vi "Calc_Actuators_SP PV to Power.vi"(0 "Power IN":dbl=0.01 format="%#_13g", 3 "Setpoint":dbl format="%.1f", 4 "Process Variable":dbl format="%.1f", 7 "power rate per iter":dbl=0.01 format="%#_13g", 9 "Deadband":dbl=1.0 format="%#_13g", 11 "Limit Max":dbl format="%.1f", 13 "Limit Min":dbl format="%.1f") -> (14 "Power OUT":dbl=0.01 format="%#_13g")   [LabVIEW 2017]
uses:
  Type Definitions/typedef_enum_Actuator Action.ctl
  7370e306-27d6-4c0f-bd38-d504dbee8b0f.vi
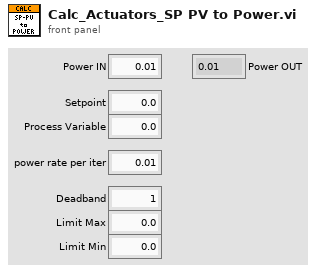
[diagram p1: front panel]
types:
  T1 = typedef "typedef_enum_Actuator Action.ctl" = enum16{"Low Limit", "Deadband", "High Limit", "Retract", "Extend"}
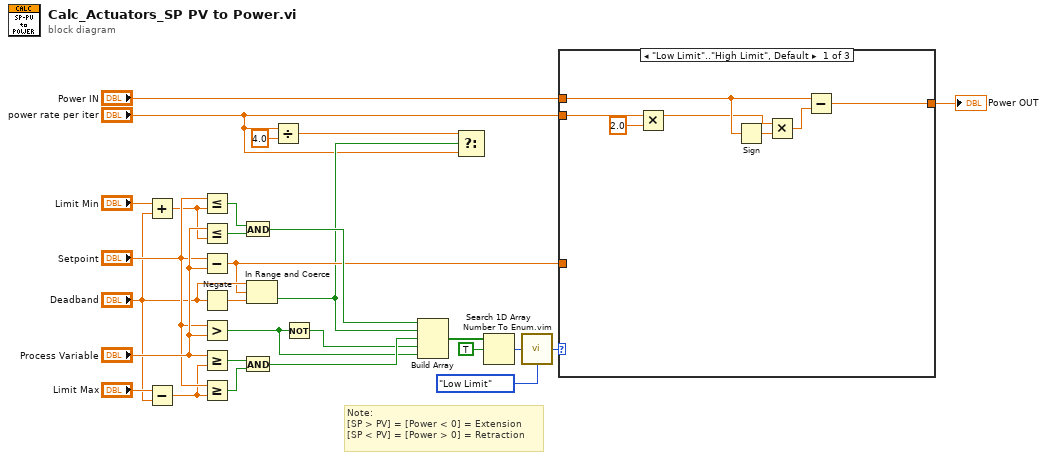
[diagram p0: block diagram]
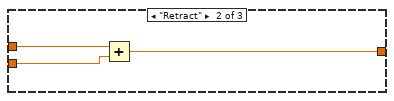
[diagram p2: hidden frame]
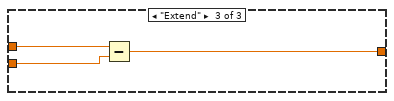
[diagram p3: hidden frame]
diagram:
  # "Note:\n[SP > PV] = [Power < 0] = Extension\n[SP < PV] = [Power > 0] = Retraction"
  n1 = Add(x="Limit Min", y="Deadband") -> (x+y=w10:dbl)
  n2 = Subtract(x="Limit Max", y="Deadband") -> (x-y=w11:dbl)
  n3 = Less Or Equal?(x="Setpoint", y=w10) -> (x <= y?=w16:bool)
  n4 = Less Or Equal?(x="Process Variable", y=w10) -> (x <= y?=w24:bool)
  n5 = Subtract(x="Setpoint", y="Process Variable") -> (x-y=w6:dbl)
  n6 = Negate(x="Deadband") -> (-x=w26:dbl)
  n7 = Greater?(x="Setpoint", y="Process Variable") -> (0:w3:bool)
  n8 = Greater Or Equal?(x="Process Variable", y=w11) -> (x >= y?=w23:bool)
  n9 = Greater Or Equal?(x="Setpoint", y=w11) -> (x >= y?=w13:bool)
  n10 = And(x=w16, y=w24) -> (x .and. y?=w17:bool)
  n11 = And(x=w23, y=w13) -> (x .and. y?=w4:bool)
  n12 = In Range and Coerce(upper limit="Deadband", x=w6, lower limit=w26) -> (In Range?=w5:bool)  [unwired: 1 out]
  n13 = Divide(x="power rate per iter", y=4.0) -> (x/y=w7:dbl)
  n14 = Not(x=w3) -> (.not. x?=w2:bool)
  n15 = Build Array(w17, w5, w4, w2, w3) -> (w22:bool[])
  n16 = Select(t=w7, s=w5, f="power rate per iter") -> ()  [unwired: 1 out]
  n17 = Search 1D Array(1D array=w22, element=TRUE) -> (index of element=w19:i32)  [unwired: 1 in]
  n18 = call "Number To Enum.vim"("number"=w19, "enum type"=typedef_enum_Actuator_Action."Low Limit" ("t")) -> ("number as enum"=w18:T1)
  n19 = case shown="\"Low Limit\"..\"High Limit\", Default" w18 {
    tunnel: "power rate per iter" -> [w34 w37 w40]
    tunnel: "Power IN" -> [w33 w38 w41]
    tunnel: [w31 w36 w39] -> w12
    tunnel: w6 -> [_ _ _]
    frame "Low Limit".."High Limit", Default {
      n20 = Multiply(x=w34, y=2.0) -> (x*y=w30:dbl)
      n21 = Sign(1:w33) -> (0:w35:dbl)
      n22 = Multiply(x=w30, y=w35) -> (x*y=w32:dbl)
      n23 = Subtract(x=w33, y=w32) -> (x-y=w31:dbl)
    }
    frame "Retract" {
      n24 = Add(x=w38, y=w37) -> (x+y=w36:dbl)
    }
    frame "Extend" {
      n25 = Subtract(x=w41, y=w40) -> (x-y=w39:dbl)
    }
  }
  "Power OUT" <- w12
